vi "Hessenberg Decomposition.vi"   [LabVIEW 2020, in "NI_AALPro.lvlib"]
doc: "Performs the Hessenberg decomposition of <B>Input Matrix</B>. Wire data to the <B>Input Matrix</B> input to determine the polymorphic instance to use or manually select the instance."
uses:
  NI_AALPro.lvlib
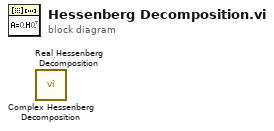
[diagram p0: block diagram]
diagram:
  n1 = call "Complex Hessenberg Decomposition.vi"() -> ()  [unwired: 9 in, 3 out]
  n2 = call "Real Hessenberg Decomposition.vi"() -> ()  [unwired: 9 in, 3 out]
